vi "e.gate HighSpeedPort Delete File.vi"(8 "error in (no error)":errorcluster, 9 "Timeout":i32, 10 "FileName":string="\u0000\t\f\u0000\u0000\u0000\u0000", 11 "Configuration in":T1 {"StartTime" format="%#.10f"; "dActTimeToSecondFactor" format="%#.10f"; "StartTimeToDayFactor" format="%#_10f"}) -> (0 "error IO":errorcluster)   [LabVIEW 2013]
uses:
  e.gate Configuration.ctl
  e.gate Channel Data.ctl
  e.gate Data Type.ctl
  e.gate Protocol Type.ctl
  e.gate Module  Data.ctl
  e.gateHSP_DLLhandle.ctl
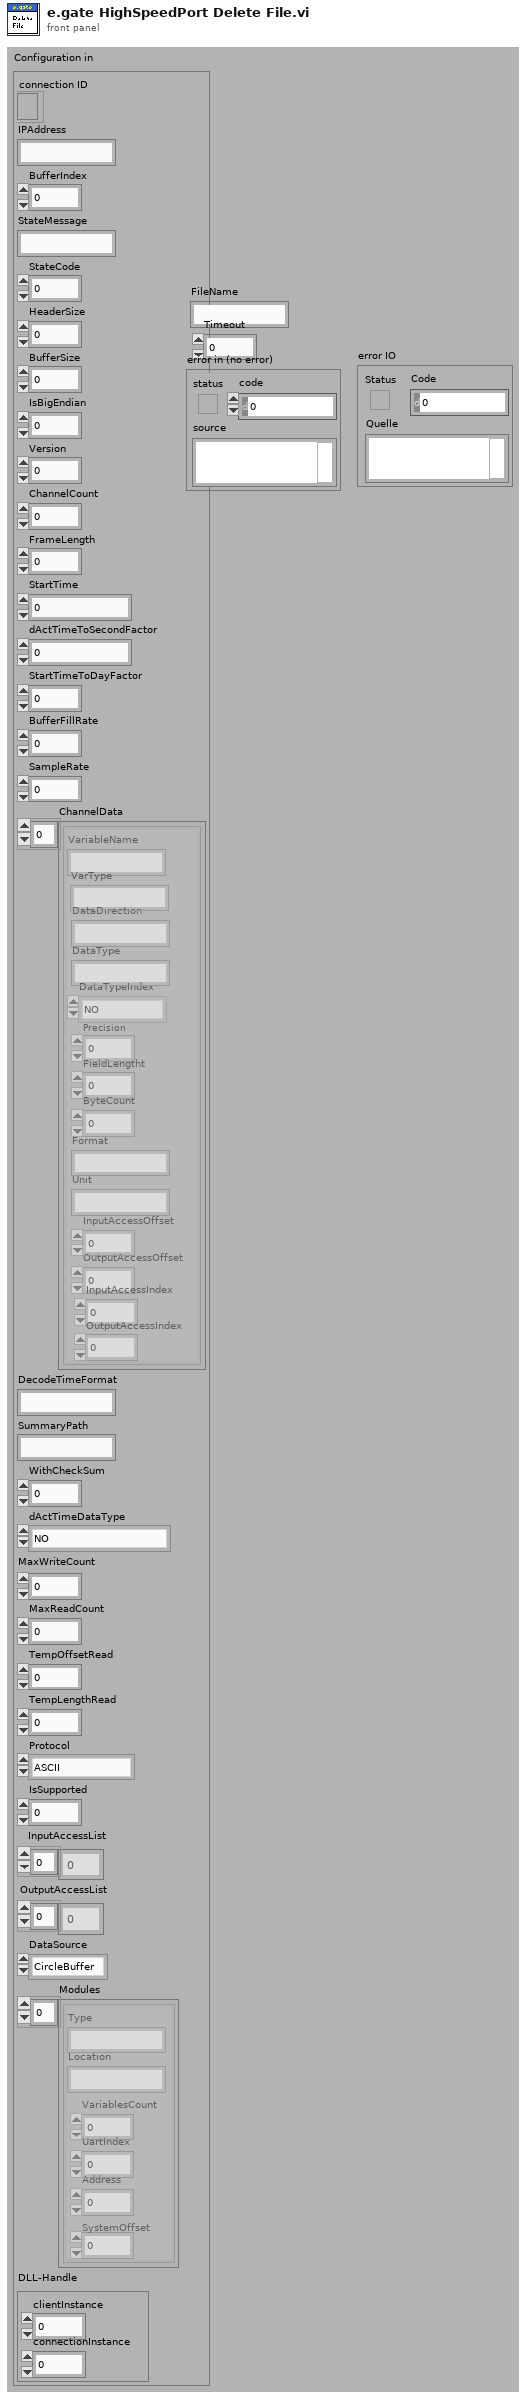
[diagram p1: front panel]
types:
  T1 = typedef "e.gate Configuration.ctl" = cluster{"connection ID":refnum<k5>, "IPAddress":string, "BufferIndex":i32, "StateMessage":string, "StateCode":i8, "HeaderSize":i32, "BufferSize":i32, "IsBigEndian":i32, "Version":i32, "ChannelCount":i32, "FrameLength":i32, "StartTime":dbl, "dActTimeToSecondFactor":dbl, "StartTimeToDayFactor":dbl, "BufferFillRate":dbl, "SampleRate":dbl, "ChannelData":T2[], "DecodeTimeFormat":string, "SummaryPath":string, "WithCheckSum":i32, "dActTimeDataType":T3, "MaxWriteCount":i32, "MaxReadCount":i32, "TempOffsetRead":i32, "TempLengthRead":i32, "Protocol":T4, "IsSupported":i32, "InputAccessList":i32[], "OutputAccessList":i32[], "DataSource":enum16{"CircleBuffer", "test.con Logger", "test.con Archive"}, "Modules":T5[], "DLL-Handle":T6}
  T2 = typedef "e.gate Channel Data.ctl" = cluster{"VariableName":string, "DataDirection":string, "DataType":string, "DataTypeIndex":T3, "Precision":i16, "FieldLengtht":i16, "ByteCount":i32, "Format":string, "Unit":string, "InputAccessOffset":i32, "OutputAccessOffset":i16, "InputAccessIndex":i16, "OutputAccessIndex":i16, "VarType":string}
  T3 = typedef "e.gate Data Type.ctl" = enum16{"NO", "BOOL", "SINT8", "USINT8", "SINT16", "USINT16", "SINT32", "USINT32", "FLOAT", "SET8", "SET16", "SET32", "DOUBLE", "SINT64", "USINT64", "SET64"}
  T4 = typedef "e.gate Protocol Type.ctl" = enum16{"ASCII", "HighspeedPort Online", "HighspeedPort Buffer", "eGateHighspeedPortDLL "}
  T5 = typedef "e.gate Module  Data.ctl" = cluster{"Type":string, "Location":string, "VariablesCount":i16, "UartIndex":i16, "Address":i16, "SystemOffset":i16}
  T6 = typedef "e.gateHSP_DLLhandle.ctl" = cluster{"clientInstance":i32, "connectionInstance":i32}
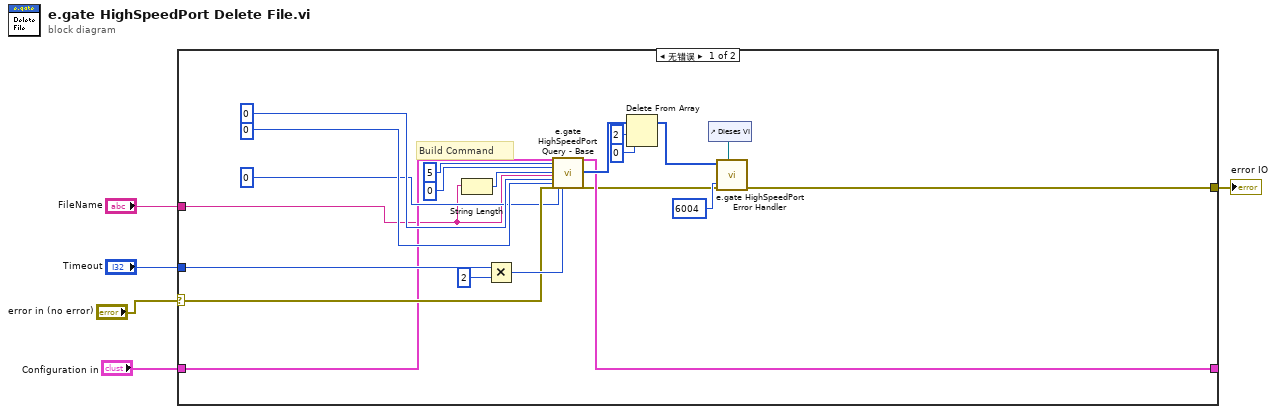
[diagram p0: block diagram]
diagram:
  n1 = case shown="无错误" "error in (no error)" {
    selector: "error in (no error)" -> [w20 w27]
    tunnel: [w12 w28] -> _
    tunnel: "Configuration in" -> [w13 w28]
    tunnel: [w6 w27] -> w1
    tunnel: "Timeout" -> [w26 _]
    tunnel: "FileName" -> [w7 _]
    frame No Error {
      # "Build Command"
      n2 = String Length(string=w7) -> (length=w21:i32)
      n3 = Multiply(x=w26, y=2) -> (x*y=w24:i32)
      n4 = call "e.gate HighSpeedPort Query - Base.vi"("e.gate Configuration in"=w13, "Command"=5, "OffsetWrite"=0 ("Command"), "LengthWrite"=w21, "DataWrite"=w7, "OffsetRead"=0 ("Command"), "LengthRead"=0 ("Command"), "error in (no error)"=w20, "TCP LengthReadt"=0, "Timeout (1000)"=w24) -> ("e.gate Configuration out"=w12:T1, "Data (out binary)"=w16:u8[], "error out"=w8:errorcluster)  [unwired: 15 out]
      n5 = Delete From Array(array=w16, length=2, index=0) -> (array with subset deleted=w9:u8[])  [unwired: 1 out]
      n6 = control-ref of="Dieses VI"() -> (w10:refnum<vi>)
      n7 = call "e.gate HighSpeedPort Error Handler.vi"("error code start index"=6004, "VI reference"=w10, "error in (no error)"=w8, "binary data in"=w9) -> ("error out"=w6:errorcluster)  [unwired: 7 out]
    }
    frame Error {
    }
  }
  "error IO" <- w1
